vi "UUT Comms.vi"(8 "error in":errorcluster, 11 "Command":T1) -> (0 "error out":errorcluster, 1 "Vdd":dbl format="%#_g V", 2 "Temperature":dbl format="%#_g°C", 3 "received Packets":u32)   [LabVIEW 2013]
doc: "This VI will emulate comms operations to the EUT"
uses:
  UUT Control Command.ctl
  Globals/Test Criteria Global.vi
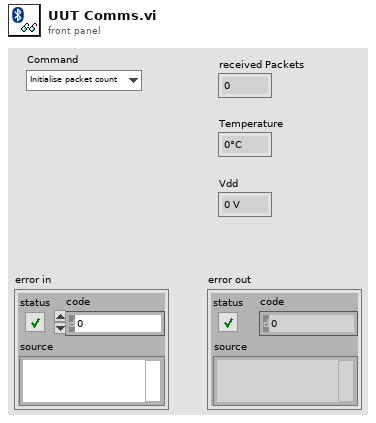
[diagram p1: front panel]
types:
  T1 = typedef "UUT Control Command.ctl" = enum16{"Initialise packet count", "Read Packet Count", "Return Temperature", "Return Operating Voltage"}
  T2 = typedef "Pass Weighting.ctl" = enum16{"Always Pass", "Always Fail", "Always 30%", "Always 31%", "Random"}
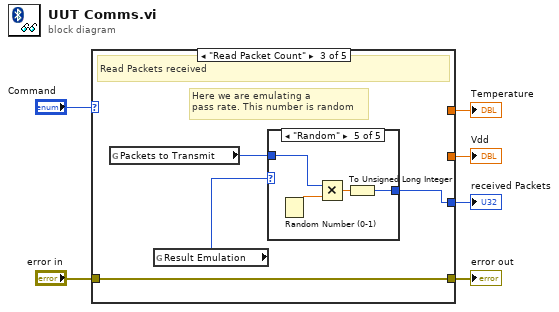
[diagram p0: block diagram]
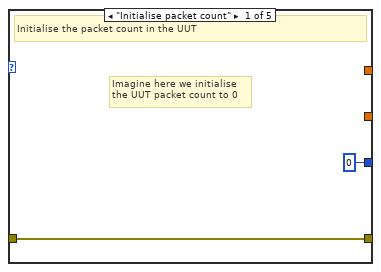
[diagram p2: hidden frame]
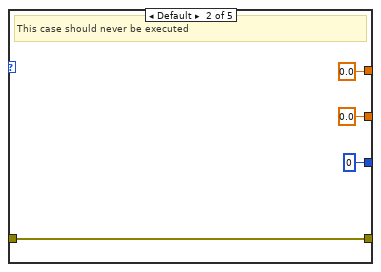
[diagram p3: hidden frame]
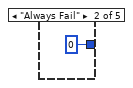
[diagram p5: hidden frame]
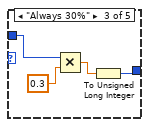
[diagram p6: hidden frame]
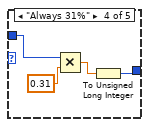
[diagram p7: hidden frame]
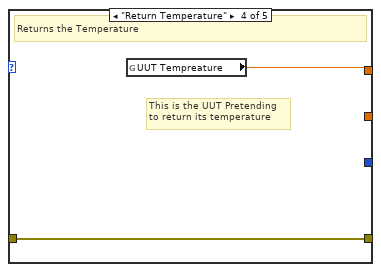
[diagram p8: hidden frame]
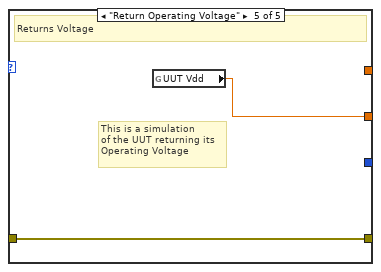
[diagram p9: hidden frame]
diagram:
  n1 = case shown="\"Read Packet Count\"" "Command" {
    tunnel: [u32 0 u32 0 w13 _ _] -> w5
    tunnel: [w7 w11 w15 w32 w34] -> w3
    tunnel: "error in" -> [w7 w11 w15 w32 w34]
    tunnel: [_ 0.0 _ _ w33] -> w2
    tunnel: [_ 0.0 _ w31 _] -> w1
    frame "Initialise packet count" {
      # "Imagine here we initialise\nthe UUT packet count to 0"
      # "Initialise the packet count in the UUT"
    }
    frame Default {
      # "This case should never be executed"
    }
    frame "Read Packet Count" {
      # "Here we are emulating a\npass rate. This number is random"
      # "Read Packets received"
      n2 = global read "Test Criteria Global.vi" "Packets to Transmit"() -> (w16:u32)
      n3 = global read "Test Criteria Global.vi" "Result Emulation"() -> (w14:T2)
      n4 = case shown="\"Random\"" w14 {
        tunnel: w16 -> [w17 _ w22 w26 w30]
        tunnel: [w17 u32 0 ("Packets to Transmit") w20 w24 w27] -> w13
        frame "Always Pass", Default {
        }
        frame "Always Fail" {
        }
        frame "Always 30%" {
          n5 = Multiply(x=w22, y=0.3) -> (x*y=w19:dbl)
          n6 = To Unsigned Long Integer(number=w19) -> (unsigned 32bit integer=w20:u32)
        }
        frame "Always 31%" {
          n7 = Multiply(x=w26, y=0.31) -> (x*y=w23:dbl)
          n8 = To Unsigned Long Integer(number=w23) -> (unsigned 32bit integer=w24:u32)
        }
        frame "Random" {
          n9 = Random Number (0-1)() -> (number: 0 to 1=w29:dbl)
          n10 = Multiply(x=w30, y=w29) -> (x*y=w28:dbl)
          n11 = To Unsigned Long Integer(number=w28) -> (unsigned 32bit integer=w27:u32)
        }
      }
    }
    frame "Return Temperature" {
      # "This is the UUT Pretending\nto return its temperature"
      # "Returns the Temperature"
      n12 = global read "Test Criteria Global.vi" "UUT Tempreature"() -> (w31:dbl)
    }
    frame "Return Operating Voltage" {
      # "This is a simulation\nof the UUT returning its\nOperating Voltage"
      # "Returns Voltage"
      n13 = global read "Test Criteria Global.vi" "UUT Vdd"() -> (w33:dbl)
    }
  }
  "received Packets" <- w5
  "error out" <- w3
  "Temperature" <- w1
  "Vdd" <- w2
